vi "Draw Steering Frame Picture.vi"(6 "steering frame position":T1, 7 "drawing options":T2={"draw wheel states?"=FALSE, "highlight wheel index"=-1, "pixels per unit"=10.0, "draw forward velocity?"=FALSE, "velocity scale"=1.0}, 8 "error in (no error)":errorcluster, 9 "picture draw area size (pixels)":cluster{"width":u32, "height":u32}={"width"=500, "height"=500}, 10 "picture in":picture, 11 "steering frame in":refnum<class "NI_Robotics_Steering Frame.lvclass">) -> (0 "error out":errorcluster, 2 "picture out":picture, 3 "steering frame out":refnum<class "NI_Robotics_Steering Frame.lvclass">)   [LabVIEW 2017, in "NI_Robotics_Steering Picture.lvlib"]
doc: "Creates an image you can wire to a 2D picture control to visualize a steering frame on the front panel. The picture can display data about the directions and velocities at which wheels move."
uses:
  <vilib>/robotics/Utilities/Visualization/Steering Visualization/Steering Picture/NI_Robotics_Steering Picture.lvlib
  <vilib>/robotics/Steering/Steering Frame/NI_Robotics_Steering Frame.lvclass
  <vilib>/robotics/Utilities/Visualization/Steering Visualization/Steering Picture/Draw Steering Frame Options.ctl
  <vilib>/robotics/Utilities/Visualization/Steering Visualization/Steering Picture/Picture Info.ctl
  <vilib>/Utility/miscctls.llb/LVBoundsTypeDef.ctl
  <vilib>/robotics/Steering/Steering Frame/NI_Robotics_Steering Frame.lvclass/NI_Robotics_Steering Frame.ctl
  <vilib>/Analysis/coordinate.llb/2D Cartesian Coordinate Rotation (Array).vi
  <vilib>/Analysis/coordinate.llb/Angle Rotation with Same Angle (array).vi
  <vilib>/robotics/Utilities/Visualization/Steering Visualization/Steering Picture/Draw Arrow.vi
  <vilib>/robotics/Utilities/Visualization/Steering Visualization/Steering Picture/Draw Wheel Axle.vi
  <vilib>/robotics/Utilities/Visualization/Steering Visualization/Steering Picture/Draw Wheel Outline.vi
  <vilib>/robotics/Utilities/Visualization/Steering Visualization/Steering Picture/Draw Fixed Wheel Forward Velocity.vi
  <vilib>/robotics/Utilities/Visualization/Steering Visualization/Steering Picture/Draw Wedge.vi
  <vilib>/robotics/Utilities/Visualization/Steering Visualization/Steering Picture/Draw Steering Wheel Forward Velocity.vi
  <vilib>/Analysis/coordinate.llb/Angle Rotation (scalar).vi
  <vilib>/Analysis/coordinate.llb/2D Cartesian Coordinate Rotation (Scalar).vi
  <vilib>/robotics/Utilities/Visualization/Steering Visualization/Steering Picture/Global Position to Pixel.vi
  <vilib>/robotics/Utilities/Visualization/Steering Visualization/Steering Picture/Draw Caster Wheel Forward Velocity.vi
  <vilib>/robotics/Utilities/Visualization/Steering Visualization/Steering Picture/Draw Lines.vi
  <vilib>/Analysis/coordinate.llb/Wrap Angle (array).vi
  <vilib>/Analysis/coordinate.llb/Wrap Angle.vi
  <vilib>/Analysis/coordinate.llb/Wrap Angle (scalar).vi
  <vilib>/picture/picture.llb/Draw Line.vi
  <vilib>/picture/picture.llb/Move Pen.vi
  <vilib>/picture/picture.llb/Draw Point.vi
  <vilib>/picture/picture.llb/Draw Multiple Lines.vi
  <vilib>/robotics/Steering/Wheel/Get Wheel Information.vi
  <vilib>/robotics/Steering/Wheel/Get Omnidirectional Wheel Information.vi
  <vilib>/robotics/Steering/Wheel/Get Mecanum Wheel Information.vi
  <vilib>/robotics/Steering/Wheel/Get Caster Wheel Information.vi
  <vilib>/picture/pictutil.llb/Draw Circle by Radius.vi
  <vilib>/Utility/AngleManip/Radians to Degrees.vi
  <vilib>/Utility/AngleManip/Radians to Degrees (Scalar DBL).vi
  <vilib>/robotics/Steering/Wheel/Get Steering Wheel Information.vi
  <vilib>/robotics/Steering/Wheel/Get Fixed Wheel Information.vi
  <vilib>/robotics/Steering/Wheel/NI_Robotics_Wheel.lvclass
  <vilib>/Analysis/NI_AALPro.lvlib
  <vilib>/Analysis/NI_AAL_Angle.lvlib
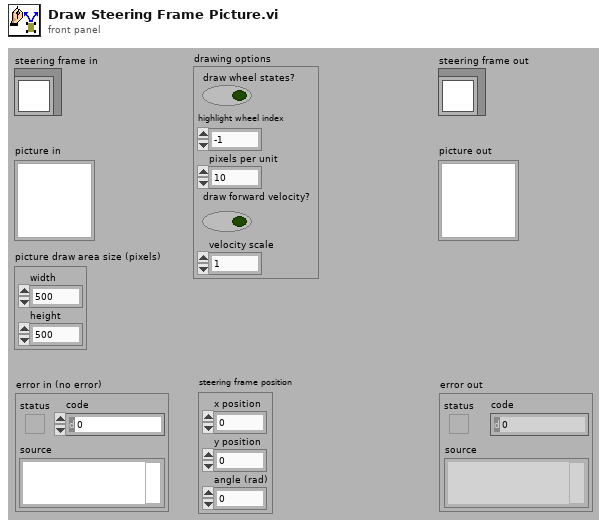
[diagram p1: front panel]
types:
  T1 = cluster{"x position":dbl, "y position":dbl, "angle (rad)":dbl}
  T2 = typedef "NI_Robotics_Steering Picture.lvlib/Draw Steering Frame Options.ctl" = cluster{"draw wheel states?":bool, "highlight wheel index":i32, "pixels per unit":dbl, "draw forward velocity?":bool, "velocity scale":dbl}
  T3 = typedef "NI_Robotics_Steering Picture.lvlib/Picture Info.ctl" = cluster{"picture size":T4, "pixels per unit":dbl}
  T4 = typedef "LVBoundsTypeDef.ctl" = cluster{"Width":u32, "Height":u32}
  T5 = typedef "NI_Robotics_Steering Picture.lvlib/Draw Wheel Options.ctl" = cluster{"global wheel position":cluster{"x":dbl, "y":dbl}, "wheel frame angle (rad)":dbl, "color (black)":u32, "draw wheel state":bool, "draw forward velocity":bool, "velocity scale":dbl, "velocity color (red)":u32}
  T6 = typedef "NI_Robotics_Wheel.lvclass/Wheel State.ctl" = cluster{"wheel name":string, "forward angular velocity":dbl, "caster angular velocity":dbl, "caster wheel angle (rad)":dbl, "steering angle (rad)":dbl}
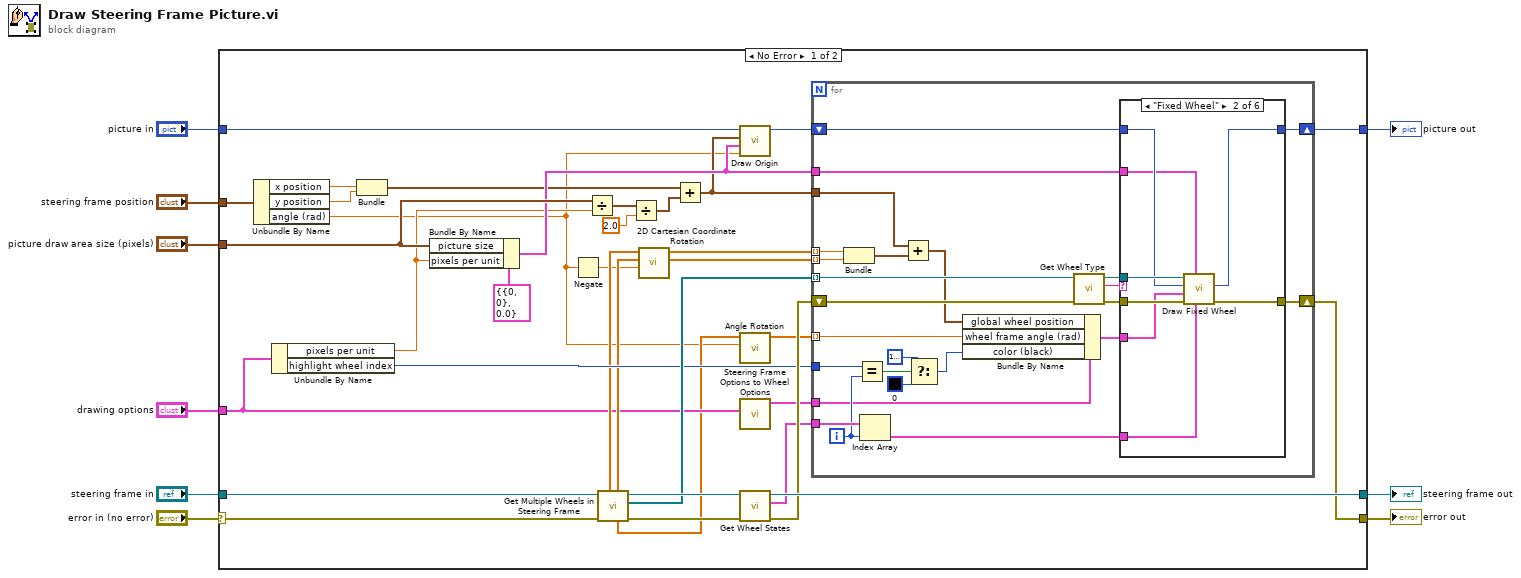
[diagram p0: block diagram]
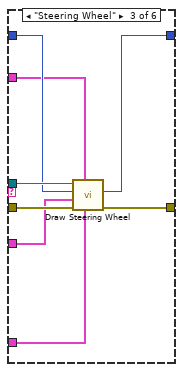
[diagram p3: hidden frame]
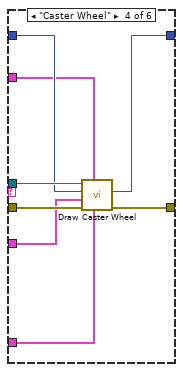
[diagram p4: hidden frame]
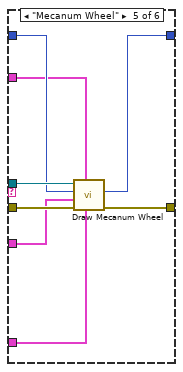
[diagram p5: hidden frame]
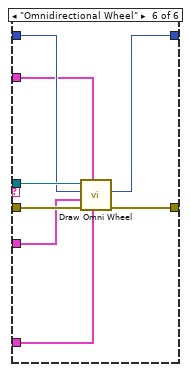
[diagram p6: hidden frame]
diagram:
  n1 = case shown="No Error" "error in (no error)" {
    selector: "error in (no error)" -> [w40 w114]
    tunnel: [w29 w114] -> w8
    tunnel: "steering frame in" -> [w42 w113]
    tunnel: [w35 w113] -> w6
    tunnel: "picture in" -> [w44 w112]
    tunnel: [w30 w112] -> w4
    tunnel: "drawing options" -> [w15 _]
    tunnel: "picture draw area size (pixels)" -> [w36 _]
    tunnel: "steering frame position" -> [w19 _]
    frame No Error {
      n2 = Unbundle By Name(w19) -> ("x position"=w18:dbl, "y position"=w17:dbl, "angle (rad)"=w11:dbl)
      n3 = Unbundle By Name(w15) -> ("pixels per unit"=w13:dbl, "highlight wheel index"=w31:i32)
      n4 = Bundle("x position"=w18, "y position"=w17) -> (w16:cluster{"x position":dbl, "y position":dbl})  [unwired: 1 in]
      n5 = Bundle By Name(cluster=T3 {"picture size"={"Width"=0, "Height"=0}, "pixels per unit"=0.0} ("picture info"), "picture size"=w36, "pixels per unit"=w13) -> (w27:T3)
      n6 = Negate(x=w11) -> (-x=w20:dbl)
      n7 = Divide(x=w36, y=w13) -> (x/y=w37:cluster{"width":dbl, "height":dbl})
      n8 = call <vilib>:"Get Multiple Wheels in Steering Frame.vi"("error in (no error)"=w40, "steering frame in"=w42) -> ("error out"=w39:errorcluster, "wheels"=w32:refnum<class "NI_Robotics_Wheel.lvclass">[], "steering frame out"=w41:refnum<class "NI_Robotics_Steering Frame.lvclass">, "frame angles (rad)"=w12:dbl[], "y positions"=w22:dbl[], "x positions"=w24:dbl[])  [unwired: 3 in, 1 out]
      n9 = Divide(x=w37, y=2.0) -> (x/y=w26:cluster{"width":dbl, "height":dbl})
      n10 = call-poly <vilib>:"2D Cartesian Coordinate Rotation.vi"("theta"=w20, "Y"=w22, "X"=w24) -> ("Y Out"=w21:dbl[], "X Out"=w23:dbl[])  [unwired: 6 in, 1 out]
      n11 = Add(x=w16, y=w26) -> (x+y=w25:cluster{dbl, dbl})
      n12 = call <vilib>:"Draw Origin.vi"("frame angle (rad)"=w11, "picture info"=w27, "frame offset position"=w25, "picture in"=w44) -> ("picture out"=w28:picture)  [unwired: 7 in]
      n13 = call-poly <vilib>:"Angle Rotation.vi"("counterclockwise rotation"=w11, "Angle"=w12) -> ("Rotated Angle"=w10:dbl[])  [unwired: 8 in, 1 out]
      n14 = call <vilib>:"Steering Frame Options to Wheel Options.vi"("draw steering frame options"=w15) -> ("draw wheel options out"=w14:T5)  [unwired: 10 in]
      n15 = call <vilib>:"Get Wheel States.vi"("error in (no error)"=w39, "steering frame in"=w41) -> ("error out"=w34:errorcluster, "wheel states"=w33:T6[], "steering frame out"=w35:refnum<class "NI_Robotics_Steering Frame.lvclass">)  [unwired: 7 in]
      n16 = for {
        tunnel: w32 -> [w69] mode=indexing
        shift-right: [w53] -> w29
        shift-left: w34 -> [w68]
        tunnel: w21 -> [w61] mode=indexing
        tunnel: w23 -> [w62] mode=indexing
        shift-right: [w63] -> w30
        shift-left: w28 -> [w64]
        tunnel: w10 -> [w47] mode=indexing
        tunnel: w25 -> [w60]
        tunnel: w27 -> [w58]
        tunnel: w31 -> [w57]
        tunnel: w33 -> [w52]
        tunnel: w14 -> [w45]
        i -> [w51]
        n17 = Bundle("Numeric"=w62, "Numeric"=w61) -> (w59:cluster{"Numeric":dbl, "Numeric":dbl})  [unwired: 1 in]
        n18 = Equal?(x=w57, y=w51) -> (x = y?=w56:bool)
        n19 = Index Array(array=w52, index=w51) -> (element=w50:T6)
        n20 = Add(x=w60, y=w59) -> (x+y=w48:cluster{dbl, dbl})
        n21 = Select(t=u32 16777224 ("color (black)"), s=w56, f=u32 0 ("color (black)")) -> (s? t:f=w46:u32)
        n22 = Bundle By Name(cluster=w45, "global wheel position"=w48, "wheel frame angle (rad)"=w47, "color (black)"=w46) -> (w49:T5)
        n23 = call-dynamic "Get Wheel Type.vi"("error in (no error)"=w68, "wheel in"=w69) -> ("error out"=w66:errorcluster, "wheel type"=w67:string, "wheel out"=w65:refnum<class "NI_Robotics_Wheel.lvclass">)  [unwired: 7 in]
        n24 = case shown="\"Fixed Wheel\"" w67 {
          tunnel: w66 -> [w70 w79 w87 w95 w103 w111]
          tunnel: w65 -> [_ w77 w85 w93 w101 w109]
          tunnel: w64 -> [w71 w76 w84 w92 w100 w108]
          tunnel: [w71 w75 w83 w91 w99 w107] -> w63
          tunnel: [w70 w78 w86 w94 w102 w110] -> w53
          tunnel: w58 -> [_ w74 w82 w90 w98 w106]
          tunnel: w50 -> [_ w73 w80 w89 w96 w104]
          tunnel: w49 -> [_ w72 w81 w88 w97 w105]
          frame "Wheel", Default {
          }
          frame "Fixed Wheel" {
            n25 = call <vilib>:"Draw Fixed Wheel.vi"("wheel state"=w73, "picture info"=w74, "error in (no error)"=w79, "draw wheel options"=w72, "picture in"=w76, "wheel in"=w77) -> ("error out"=w78:errorcluster, "picture out"=w75:picture)  [unwired: 3 in, 1 out]
          }
          frame "Steering Wheel" {
            n26 = call <vilib>:"Draw Steering Wheel.vi"("wheel state"=w80, "picture info"=w82, "error in (no error)"=w87, "draw wheel options"=w81, "picture in"=w84, "wheel in"=w85) -> ("error out"=w86:errorcluster, "picture out"=w83:picture)  [unwired: 3 in, 1 out]
          }
          frame "Caster Wheel" {
            n27 = call <vilib>:"Draw Caster Wheel.vi"("wheel state"=w89, "picture info"=w90, "error in (no error)"=w95, "draw wheel options"=w88, "picture in"=w92, "wheel in"=w93) -> ("error out"=w94:errorcluster, "picture out"=w91:picture)  [unwired: 3 in, 1 out]
          }
          frame "Mecanum Wheel" {
            n28 = call <vilib>:"Draw Mecanum Wheel.vi"("wheel state"=w96, "picture info"=w98, "error in (no error)"=w103, "draw wheel options"=w97, "picture in"=w100, "wheel in"=w101) -> ("error out"=w102:errorcluster, "picture out"=w99:picture)  [unwired: 3 in, 1 out]
          }
          frame "Omnidirectional Wheel" {
            n29 = call <vilib>:"Draw Omni Wheel.vi"("wheel state"=w104, "picture info"=w106, "error in (no error)"=w111, "draw wheel options"=w105, "picture in"=w108, "wheel in"=w109) -> ("error out"=w110:errorcluster, "picture out"=w107:picture)  [unwired: 3 in, 1 out]
          }
        }
      }
    }
    frame Error {
    }
  }
  "steering frame out" <- w6
  "error out" <- w8
  "picture out" <- w4
